vi "UsrProfiles-Window.vi"(8 "error in (no error)":errorcluster, 10 "Access source":T1(ring)) -> (0 "error out":errorcluster, 2 "Profile change":bool)   [LabVIEW 2013]
uses:
  Typedefs/User login window refs.ctl
  Global Variables/General Globals.vi
panel:
  out "error out 2":errorcluster
  in  "Users":i32(listbox)
  in  "Profiles":i32(listbox) caption="User 1's profiles"
  out "Last used":string
  in  "Load":bool
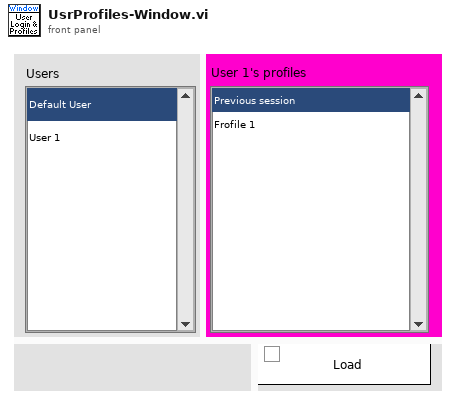
[diagram p1: front panel]
types:
  T1 = enum16{"Software Init", "User menu", "Switch User button"}
  T2 = typedef "User login window refs.ctl" = cluster{"User profiles window ref":refnum<k9>, "Users listbox":refnum<vi>, "Profiles listbox":refnum<vi>, "Last used":refnum<vi>}
  T3 = typedef "LVPoint32TypeDef.ctl" = cluster{"Horizontal":i32, "Vertical":i32}
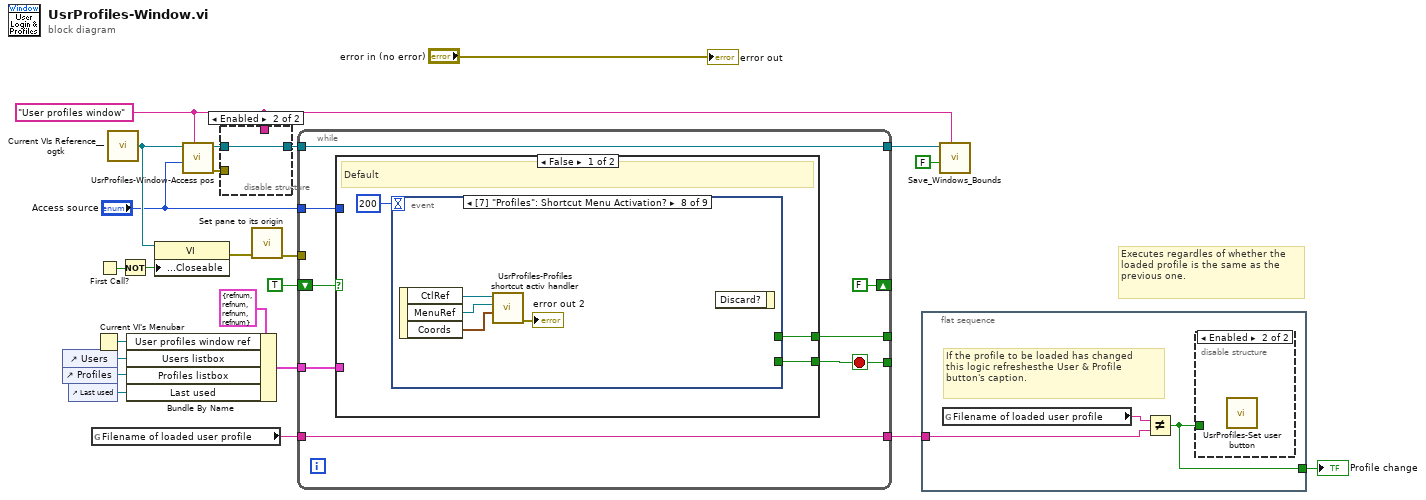
[diagram p0: block diagram]
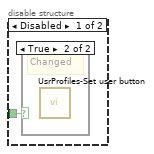
[diagram p2: hidden frame]
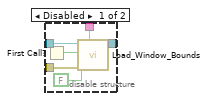
[diagram p4: hidden frame]
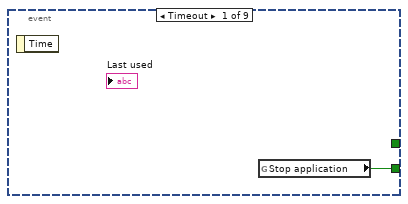
[diagram p5: hidden frame]
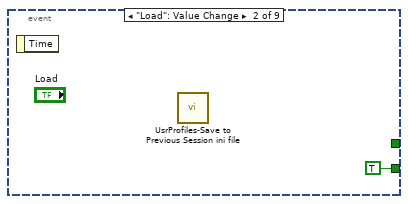
[diagram p6: hidden frame]
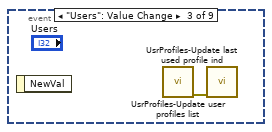
[diagram p7: hidden frame]
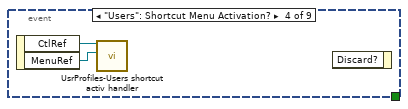
[diagram p8: hidden frame]
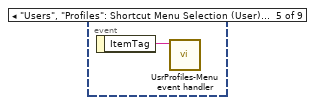
[diagram p9: hidden frame]
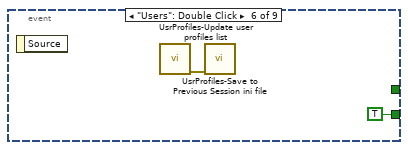
[diagram p10: hidden frame]
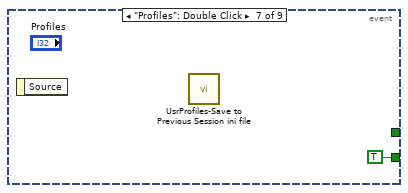
[diagram p11: hidden frame]
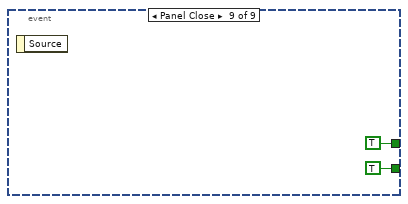
[diagram p12: hidden frame]
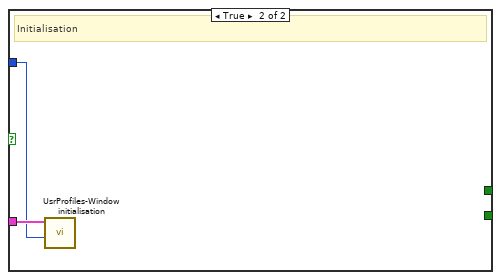
[diagram p13: hidden frame]
diagram:
  w7 = "User profiles window" ("Window Name (i.e. Key)")
  # "Executes regardles of whether the loaded profile is the same as the previous one."
  n1 = control-ref of="Users"() -> (w20:refnum<vi>)
  n2 = control-ref of="Profiles"() -> (w19:refnum<vi>)
  n3 = control-ref of="Last used"() -> (w12:refnum<vi>)
  n4 = global read "General Globals.vi" "Filename of loaded user profile"() -> (w5:string)
  n5 = Current VI's Menubar() -> (w1:refnum<k9>)
  n6 = First Call?() -> (First Call?: T/F=w11:bool)
  n7 = call "Current VIs Reference__ogtk.vi"() -> ("Current VI's reference"=w9:refnum<vi>)  [unwired: 5 in]
  n8 = Not(x=w11) -> (.not. x?=w14:bool)
  n9 = Bundle By Name(cluster=T2 {"User profiles window ref"=refnum, "Users listbox"=refnum, "Profiles listbox"=refnum, "Last used"=refnum} ("output cluster"), "User profiles window ref"=w1, "Users listbox"=w20, "Profiles listbox"=w19, "Last used"=w12) -> (w17:T2)
  n10 = property class="VI"(reference=w9, "Front Panel.Closeable"=w14) -> (error out=w13:errorcluster)  [unwired: 1 in, 1 out]
  n11 = call "UsrProfiles-Window-Access pos.vi"("Window Name"=w7, "Access source"="Access source", "VI in"=w9) -> ("error out"=w10:errorcluster, "VI out"=w8:refnum<vi>)  [unwired: 7 in]
  n12 = disable-structure shown="Enabled" {
    disable-tunnel: [w28 w30] -> w21
    disable-tunnel: w10 -> [w27 _]
    disable-tunnel: w8 -> [w26 w30]
    disable-tunnel: w7 -> [w25 _]
    frame Disabled {
      n13 = First Call?() -> (First Call?: T/F=w29:bool)
      n14 = call "Load_Window_Bounds.vi"("Window Name (i.e. Key)"=w25, "error in"=w27, "Disable"=FALSE, "First Call"=w29, "Window VI's Ref"=w26) -> ("reference out"=w28:refnum<vi>)  [unwired: 3 in, 3 out]
    }
    frame Enabled {
    }
  }
  n15 = call "Set pane to its origin.vi"("error in (no error)"=w13) -> ("error out (no error)"=w23:errorcluster)  [unwired: 9 in, 1 out]
  n16 = while {
    tunnel: w23 -> [_]
    tunnel: w21 -> [w38]
    tunnel: [w38] -> w22
    tunnel: w17 -> [w37]
    shift-right: [FALSE] -> _
    shift-left: TRUE -> [w36]
    tunnel: [w34] -> _
    tunnel: [w33] -> _
    tunnel: "Access source" -> [w32]
    tunnel: w5 -> [w31]
    tunnel: [w31] -> w4
    stop <- w34 stop-if-true
    n17 = case shown="False" w36 {
      tunnel: [w41 _] -> w34
      tunnel: w37 -> [_ w58]
      tunnel: [w39 _] -> w33
      tunnel: w32 -> [_ w57]
      frame False {
        # "Default"
        n18 = event shown="[7] \"Profiles\": Shortcut Menu Activation?" {
          selector: _ -> [_ _ _ _ _ _ _ _ _]
          dyn-events: _ -> [_ _ _ _ _ _ _ _ _]
          timeout: 200 -> [_ _ _ _ _ _ _ _ _]
          tunnel: [w42 TRUE _ _ _ TRUE ("Stop application") TRUE ("Stop application") _ TRUE] -> w41
          tunnel: [_ _ _ _ _ _ _ _ TRUE] -> w39
          event Timeout {
            n19 = event-data() -> ()  [unwired: 1 in, 1 out]
            n20 = global read "General Globals.vi" "Stop application"() -> (w42:bool)
          }
          event "Load": Value Change {
            n21 = event-data() -> ()  [unwired: 1 in, 1 out]
            n22 = call "UsrProfiles-Save to Previous Session ini file.vi"() -> ()  [unwired: 12 in]
          }
          event "Users": Value Change {
            n23 = event-data() -> ()  [unwired: 1 in, 1 out]
            n24 = call "UsrProfiles-Update user profiles list.vi"() -> ("error out"=w44:errorcluster)  [unwired: 11 in]
            n25 = call "UsrProfiles-Update last used profile ind.vi"("error in"=w44) -> ()  [unwired: 10 in, 1 out]
          }
          event "Users": Shortcut Menu Activation? {
            n26 = event-data() -> ("CtlRef"=w45:refnum<vi>, "MenuRef"=w46:refnum<k9>)  [unwired: 1 in]
            n27 = call "UsrProfiles-Users shortcut activ handler.vi"("Users ListBox MenuRef"=w46, "Users ListBox ref"=w45) -> ()  [unwired: 10 in]
            n28 = event-data() -> ()  [unwired: 2 in, 1 out]
          }
          event "Users", "Profiles": Shortcut Menu Selection (User); Menu Selection (User) {
            n29 = event-data() -> ("ItemTag"=w47:string)  [unwired: 1 in]
            n30 = call "UsrProfiles-Menu event handler.vi"("ItemTag"=w47) -> ()  [unwired: 11 in]
          }
          event "Users": Double Click {
            n31 = event-data() -> ()  [unwired: 1 in, 1 out]
            n32 = call "UsrProfiles-Update user profiles list.vi"() -> ("error out"=w48:errorcluster)  [unwired: 11 in]
            n33 = call "UsrProfiles-Save to Previous Session ini file.vi"("error in"=w48) -> ()  [unwired: 11 in]
          }
          event "Profiles": Double Click {
            n34 = event-data() -> ()  [unwired: 1 in, 1 out]
            n35 = call "UsrProfiles-Save to Previous Session ini file.vi"() -> ()  [unwired: 12 in]
          }
          event "Profiles": Shortcut Menu Activation? {
            n36 = event-data() -> ("CtlRef"=w54:refnum<vi>, "MenuRef"=w53:refnum<k9>, "Coords"=w52:T3)  [unwired: 1 in]
            n37 = call "UsrProfiles-Profiles shortcut activ handler.vi"("Coords"=w52, "Users ListBox MenuRef"=w53, "Users ListBox ref"=w54) -> ("error out"=→"error out 2":errorcluster)  [unwired: 8 in]
            n38 = event-data() -> ()  [unwired: 2 in, 1 out]
          }
          event Panel Close {
            n39 = event-data() -> ()  [unwired: 1 in, 1 out]
          }
        }
      }
      frame True {
        # "Initialisation"
        n40 = call "UsrProfiles-Window initialisation.vi"("Access source"=w57, "ctrl refs"=w58) -> ()  [unwired: 10 in]
      }
    }
  }
  n41 = flat-sequence {
    tunnel: w4 -> [w61]
    tunnel: [w59] -> w3
    frame #0 {
      # "If the profile to be loaded has changed\nthis logic refreshesthe User & Profile button's caption."
      n42 = global read "General Globals.vi" "Filename of loaded user profile"() -> (w60:string)
      n43 = Not Equal?(x=w60, y=w61) -> (x != y?=w59:bool)
      n44 = disable-structure shown="Enabled" {
        disable-tunnel: w59 -> [w62 _]
        frame Disabled {
          n45 = case shown="True" w62 {
            frame False {
              # "No change"
            }
            frame True {
              # "Changed"
              n46 = call "UsrProfiles-Set user button.vi"() -> ()  [unwired: 11 in, 1 out]
            }
          }
        }
        frame Enabled {
          n47 = call "UsrProfiles-Set user button.vi"() -> ()  [unwired: 11 in, 1 out]
        }
      }
    }
  }
  n48 = call "Save_Windows_Bounds.vi"("Window Name (i.e. Key)"=w7, "Front Panel Window:Open"=FALSE, "Window VI's Ref"=w22) -> ()  [unwired: 8 in, 1 out]
  "error out" <- "error in (no error)"
  "Profile change" <- w3
